vi "Resize To Array.vi"(9 "New Size (In)":i32, 10 "Draw Area Size (In)":T1, 11 "Picture (In)":picture) -> (3 "Image Array (Out)":u8[][](array[numeric]))   [LabVIEW 2016]
uses:
  <vilib>/Utility/miscctls.llb/LVBoundsTypeDef.ctl
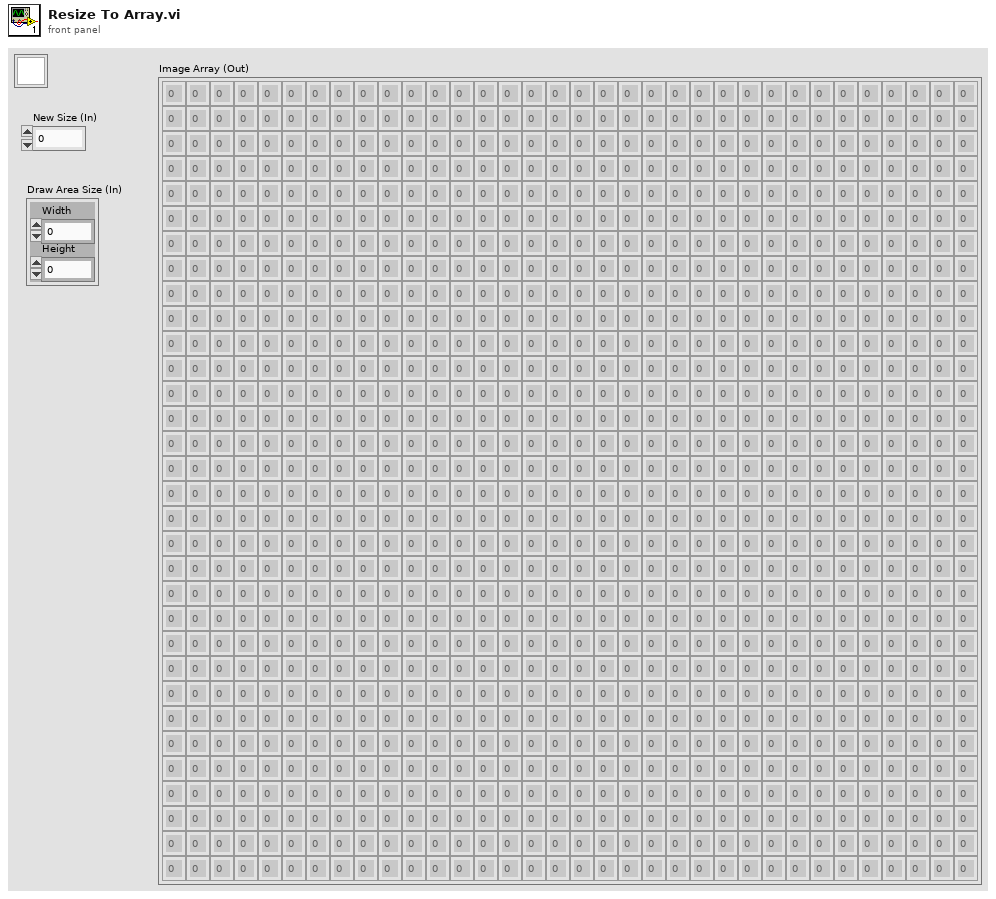
[diagram p1: front panel]
types:
  T1 = typedef "LVBoundsTypeDef.ctl" = cluster{"Width":u32, "Height":u32}
  T2 = cluster{"New Size (In)":i32, "New Size (In)":i32}
  T3 = typedef "imagedata.ctl" = cluster{"image type":i32, "image depth":i32, "image":u8[], "mask":u8[], "colors":u32[], "Rectangle":cluster{"left":i16, "top":i16, "right":i16, "bottom":i16}}
  T4 = cluster{"left":i16, "top":i16, "right":i16, "bottom":i16}
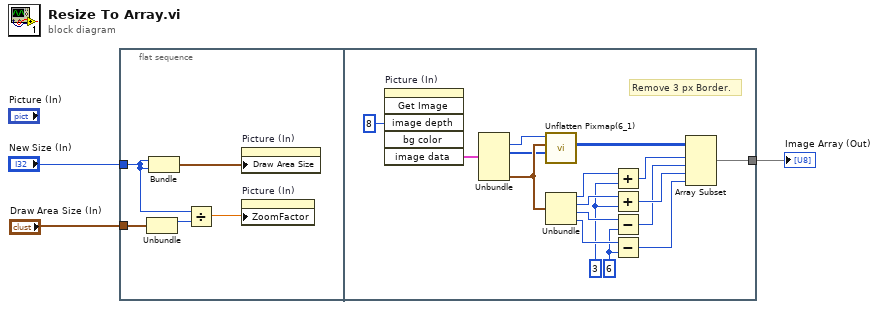
[diagram p0: block diagram]
diagram:
  n1 = flat-sequence {
    tunnel: "New Size (In)" -> [w4]
    tunnel: "Draw Area Size (In)" -> [w5]
    tunnel: [w11] -> w1
    frame #0 {
      n2 = Unbundle(w5) -> ("Width"=w8:u32)  [unwired: 1 out]
      n3 = Bundle("New Size (In)"=w4, "New Size (In)"=w4) -> (w6:T2)  [unwired: 1 in]
      n4 = Divide(x=w4, y=w8) -> (x/y=w7:dbl)
      n5 = property on="Picture (In)" class="Pict"("Draw Area Size"=w6) -> ()  [unwired: 2 in, 2 out]
      n6 = property on="Picture (In)" class="Pict"("ZoomFactor"=w7) -> ()  [unwired: 2 in, 2 out]
    }
    frame #1 {
      w10 = 3 ("Image Depth")
      w9 = 6 ("Image Depth")
      # "Remove 3 px Border."
      n7 = invoke on="Picture (In)" class="Pict" method="Get Image"("image depth"=8 ("Image Depth")) -> ("image data"=w24:T3)  [unwired: 5 in, 5 out]
      n8 = Unbundle(w24) -> ("image depth"=w23:i32, "image"=w12:u8[], "Rectangle"=w13:T4)  [unwired: 3 out]
      n9 = call <vilib>:"Unflatten Pixmap(6_1).vi"("flattened image data"=w12, "rect"=w13, "depth"=w23) -> ("8-bit pixmap"=w18:u8[][])  [unwired: 4 in, 4 out]
      n10 = Unbundle(w13) -> ("left"=w14:i16, "top"=w15:i16, "right"=w16:i16, "bottom"=w17:i16)
      n11 = Add(x=w14, y=w10) -> (x+y=w19:i32)
      n12 = Add(x=w15, y=w10) -> (x+y=w22:i32)
      n13 = Subtract(x=w16, y=w9) -> (x-y=w21:i32)
      n14 = Subtract(x=w17, y=w9) -> (x-y=w20:i32)
      n15 = Array Subset(array=w18, index (row)=w19, length (row)=w21, index (col)=w22, length (col)=w20) -> (w11:u8[][])
    }
  }
  "Image Array (Out)" <- w1
